vi "HFRR ADV v06.vi"() -> ()   [LabVIEW 2025] (continued)
              n1765 = Fract/Exp String To Number(string=w2180) -> (number=w2183:dbl)  [unwired: 3 in, 1 out]
              n1766 = Add(x=w2183, y=0.0) -> (x+y=w2179:dbl)
            }
            n1767 = for {
              N: w2071 -> [_]
              tunnel: w2078 -> [w2126]
              tunnel: w2077 -> [w2125]
              tunnel: [w2115] -> w2031 mode=indexing
              tunnel: [w2114] -> w2024 mode=indexing
              tunnel: w2068 -> [_]
              tunnel: [w2103] -> w2029 mode=indexing
              tunnel: [w2108] -> w2026 mode=indexing
              tunnel: [w2104] -> w2016 mode=indexing
              tunnel: [w2099] -> w1991 mode=indexing
              tunnel: [w2095] -> w1972 mode=indexing
              tunnel: [w2090] -> w1932 mode=indexing
              (unwired) 1.0 ("x")
              (unwired) TRUE ("line mode (F)")
              n1768 = Read from Text File "Read File"(file (use dialog)=w2126, error in=w2125) -> (text=w2091:string)  [unwired: 2 in, 3 out]
              n1769 = local write "String 12"(w2091) -> ()
              n1770 = String Subset(string=w2091, offset (0)=85, length (rest)=9 ("length (rest)")) -> (substring=w2093:string)
              n1771 = String Subset(string=w2091, offset (0)=35, length (rest)=9 ("length (rest)")) -> (substring=w2116:string)
              n1772 = String Subset(string=w2091, offset (0)=55, length (rest)=9 ("length (rest)")) -> (substring=w2101:string)
              n1773 = String Subset(string=w2091, offset (0)=25, length (rest)=9 ("length (rest)")) -> (substring=w2097:string)
              n1774 = String Subset(string=w2091, offset (0)=45, length (rest)=9 ("length (rest)")) -> (substring=w2106:string)
              n1775 = String Subset(string=w2091, offset (0)=15, length (rest)=9 ("length (rest)")) -> (substring=w2122:string)
              n1776 = String Subset(string=w2091, offset (0)=0, length (rest)=14 ("length (rest)")) -> (substring=w2119:string)
              n1777 = String Subset(string=w2091, offset (0)=65, length (rest)=9 ("length (rest)")) -> (substring=w2109:string)
              n1778 = Fract/Exp String To Number(string=w2093) -> (number=w2090:dbl)  [unwired: 3 in, 1 out]
              n1779 = Fract/Exp String To Number(string=w2116) -> (number=w2114:dbl)  [unwired: 3 in, 1 out]
              n1780 = Fract/Exp String To Number(string=w2101) -> (number=w2099:dbl)  [unwired: 3 in, 1 out]
              n1781 = Fract/Exp String To Number(string=w2097) -> (number=w2095:dbl)  [unwired: 3 in, 1 out]
              n1782 = Fract/Exp String To Number(string=w2106) -> (number=w2104:dbl)  [unwired: 3 in, 1 out]
              n1783 = Fract/Exp String To Number(string=w2122) -> (number=w2103:dbl)  [unwired: 3 in, 1 out]
              n1784 = Fract/Exp String To Number(string=w2119) -> (number=w2115:dbl)  [unwired: 3 in, 1 out]
              n1785 = Fract/Exp String To Number(string=w2109) -> (number=w2112:dbl)  [unwired: 3 in, 1 out]
              n1786 = Add(x=w2112, y=0.0) -> (x+y=w2108:dbl)
            }
            n1787 = Delete From Array(array=w1974, index=0) -> (array with subset deleted=w1947:dbl[])  [unwired: 1 in, 1 out]
            n1788 = Delete From Array(array=w2037, index=0) -> (array with subset deleted=w2010:dbl[])  [unwired: 1 in, 1 out]
            n1789 = Delete From Array(array=w2017, index=0) -> (array with subset deleted=w2005:dbl[])  [unwired: 1 in, 1 out]
            n1790 = Delete From Array(array=w2035, index=0) -> (array with subset deleted=w2036:dbl[])  [unwired: 1 in, 1 out]
            n1791 = call-poly <vilib>:"Mean.vi"("X"=w1947) -> ("mean"=→"КОФ2 4":dbl)  [unwired: 1 out]
            n1792 = call-poly <vilib>:"Mean.vi"("X"=w2010) -> ("mean"=→"КОФ3":dbl)  [unwired: 1 out]
            n1793 = call-poly <vilib>:"Mean.vi"("X"=w2005) -> ("mean"=→"CP3":dbl)  [unwired: 1 out]
            n1794 = Delete From Array(array=w1999, index=0) -> (array with subset deleted=w1926:dbl[])  [unwired: 1 in, 1 out]
            n1795 = Delete From Array(array=w1938, index=0) -> (array with subset deleted=w1925:dbl[])  [unwired: 1 in, 1 out]
            n1796 = Delete From Array(array=w1978, index=0) -> (array with subset deleted=w1949:dbl[])  [unwired: 1 in, 1 out]
            n1797 = Delete From Array(array=w2056, index=0) -> (array with subset deleted=w2011:dbl[])  [unwired: 1 in, 1 out]
            n1798 = Delete From Array(array=w2022, index=0) -> (array with subset deleted=w2007:dbl[])  [unwired: 1 in, 1 out]
            "array w/ subset deleted" <- w2007
            n1799 = Delete From Array(array=w2053, index=0) -> (array with subset deleted=w2054:dbl[])  [unwired: 1 in, 1 out]
            n1800 = call-poly <vilib>:"Mean.vi"("X"=w1949) -> ("mean"=→"КОФ2 2":dbl)  [unwired: 1 out]
            n1801 = call-poly <vilib>:"Mean.vi"("X"=w2011) -> ("mean"=→"КОФ1":dbl)  [unwired: 1 out]
            n1802 = Bundle "Bundle"(w1926, w1925) -> (w1931:cluster{dbl[], dbl[]})  [unwired: 1 in]
            n1803 = Bundle "Bundle"(w1926, w2054) -> (w1918:cluster{dbl[], dbl[]})  [unwired: 1 in]
            n1804 = Delete From Array(array=w1933, index=0) -> (array with subset deleted=w1921:dbl[])  [unwired: 1 in, 1 out]
            n1805 = Delete From Array(array=w1934, index=0) -> (array with subset deleted=w1923:dbl[])  [unwired: 1 in, 1 out]
            n1806 = Delete From Array(array=w2044, index=0) -> (array with subset deleted=w2045:dbl[])  [unwired: 1 in, 1 out]
            n1807 = Delete From Array(array=w1932, index=0) -> (array with subset deleted=w1919:dbl[])  [unwired: 1 in, 1 out]
            n1808 = Delete From Array(array=w2026, index=0) -> (array with subset deleted=w2027:dbl[])  [unwired: 1 in, 1 out]
            n1809 = Delete From Array(array=w2051, index=0) -> (array with subset deleted=w1957:dbl[])  [unwired: 1 in, 1 out]
            n1810 = Delete From Array(array=w1997, index=0) -> (array with subset deleted=w1953:dbl[])  [unwired: 1 in, 1 out]
            n1811 = Delete From Array(array=w2033, index=0) -> (array with subset deleted=w1955:dbl[])  [unwired: 1 in, 1 out]
            n1812 = Delete From Array(array=w1993, index=0) -> (array with subset deleted=w1951:dbl[])  [unwired: 1 in, 1 out]
            n1813 = Delete From Array(array=w2042, index=0) -> (array with subset deleted=w1956:dbl[])  [unwired: 1 in, 1 out]
            n1814 = Delete From Array(array=w1995, index=0) -> (array with subset deleted=w1952:dbl[])  [unwired: 1 in, 1 out]
            n1815 = Delete From Array(array=w1976, index=0) -> (array with subset deleted=w1948:dbl[])  [unwired: 1 in, 1 out]
            n1816 = Delete From Array(array=w2020, index=0) -> (array with subset deleted=w2006:dbl[])  [unwired: 1 in, 1 out]
            n1817 = Delete From Array(array=w2047, index=0) -> (array with subset deleted=w2008:dbl[])  [unwired: 1 in, 1 out]
            n1818 = Delete From Array(array=w2024, index=0) -> (array with subset deleted=w1954:dbl[])  [unwired: 1 in, 1 out]
            n1819 = Delete From Array(array=w1991, index=0) -> (array with subset deleted=w1950:dbl[])  [unwired: 1 in, 1 out]
            n1820 = Delete From Array(array=w1972, index=0) -> (array with subset deleted=w1946:dbl[])  [unwired: 1 in, 1 out]
            n1821 = Delete From Array(array=w2016, index=0) -> (array with subset deleted=w2004:dbl[])  [unwired: 1 in, 1 out]
            n1822 = Delete From Array(array=w2029, index=0) -> (array with subset deleted=w2009:dbl[])  [unwired: 1 in, 1 out]
            n1823 = Delete From Array(array=w2039, index=0) -> (array with subset deleted=w1922:dbl[])  [unwired: 1 in, 1 out]
            n1824 = Delete From Array(array=w2049, index=0) -> (array with subset deleted=w1924:dbl[])  [unwired: 1 in, 1 out]
            n1825 = Delete From Array(array=w2031, index=0) -> (array with subset deleted=w1920:dbl[])  [unwired: 1 in, 1 out]
            n1826 = Bundle "Bundle"(w1926, w1957) -> (w1944:cluster{dbl[], dbl[]})  [unwired: 1 in]
            n1827 = Bundle "Bundle"(w1926, w2011) -> (w1945:cluster{dbl[], dbl[]})  [unwired: 1 in]
            n1828 = Bundle "Bundle"(w1957, w1953) -> (w1959:cluster{dbl[], dbl[]})  [unwired: 1 in]
            n1829 = Bundle "Bundle"(w1922, w1921) -> (w1929:cluster{dbl[], dbl[]})  [unwired: 1 in]
            n1830 = Bundle "Bundle"(w1955, w1951) -> (w1961:cluster{dbl[], dbl[]})  [unwired: 1 in]
            n1831 = Bundle "Bundle"(w1922, w1955) -> (w2065:cluster{dbl[], dbl[]})  [unwired: 1 in]
            n1832 = Bundle "Bundle"(w1922, w1951) -> (w1989:cluster{dbl[], dbl[]})  [unwired: 1 in]
            n1833 = Bundle "Bundle"(w1922, w2010) -> (w2075:cluster{dbl[], dbl[]})  [unwired: 1 in]
            n1834 = Bundle "Bundle"(w1922, w2005) -> (w2013:cluster{dbl[], dbl[]})  [unwired: 1 in]
            n1835 = Bundle "Bundle"(w1922, w2036) -> (w2060:cluster{dbl[], dbl[]})  [unwired: 1 in]
            n1836 = Bundle "Bundle"(w1956, w1952) -> (w1960:cluster{dbl[], dbl[]})  [unwired: 1 in]
            n1837 = Bundle "Bundle"(w1924, w1923) -> (w1930:cluster{dbl[], dbl[]})  [unwired: 1 in]
            n1838 = Bundle "Bundle"(w1924, w1956) -> (w2067:cluster{dbl[], dbl[]})  [unwired: 1 in]
            n1839 = Bundle "Bundle"(w1924, w1952) -> (w1990:cluster{dbl[], dbl[]})  [unwired: 1 in]
            n1840 = Bundle "Bundle"(w1924, w2006) -> (w2014:cluster{dbl[], dbl[]})  [unwired: 1 in]
            n1841 = Bundle "Bundle"(w1924, w2008) -> (w2076:cluster{dbl[], dbl[]})  [unwired: 1 in]
            n1842 = Bundle "Bundle"(w1924, w2045) -> (w2058:cluster{dbl[], dbl[]})  [unwired: 1 in]
            n1843 = Bundle "Bundle"(w1954, w1950) -> (w1962:cluster{dbl[], dbl[]})  [unwired: 1 in]
            n1844 = Bundle "Bundle"(w1920, w1919) -> (w1928:cluster{dbl[], dbl[]})  [unwired: 1 in]
            n1845 = Bundle "Bundle"(w1920, w1954) -> (w2066:cluster{dbl[], dbl[]})  [unwired: 1 in]
            n1846 = Bundle "Bundle"(w1920, w1950) -> (w1988:cluster{dbl[], dbl[]})  [unwired: 1 in]
            n1847 = Bundle "Bundle"(w1920, w2004) -> (w2012:cluster{dbl[], dbl[]})  [unwired: 1 in]
            n1848 = Bundle "Bundle"(w1920, w2009) -> (w2074:cluster{dbl[], dbl[]})  [unwired: 1 in]
            n1849 = Bundle "Bundle"(w1920, w2027) -> (w2059:cluster{dbl[], dbl[]})  [unwired: 1 in]
            n1850 = call-poly <vilib>:"Mean.vi"("X"=w2007) -> ("mean"=→"CP1":dbl)  [unwired: 1 out]
            n1851 = call-poly <vilib>:"Mean.vi"("X"=w1948) -> ("mean"=→"КОФ2 3":dbl)  [unwired: 1 out]
            n1852 = call-poly <vilib>:"Mean.vi"("X"=w2006) -> ("mean"=→"CP2":dbl)  [unwired: 1 out]
            n1853 = call-poly <vilib>:"Mean.vi"("X"=w2008) -> ("mean"=→"КОФ2":dbl)  [unwired: 1 out]
            n1854 = call-poly <vilib>:"Mean.vi"("X"=w1946) -> ("mean"=→"КОФ2 5":dbl)  [unwired: 1 out]
            n1855 = call-poly <vilib>:"Mean.vi"("X"=w2004) -> ("mean"=→"CP4":dbl)  [unwired: 1 out]
            n1856 = call-poly <vilib>:"Mean.vi"("X"=w2009) -> ("mean"=→"КОФ4":dbl)  [unwired: 1 out]
            n1857 = Bundle "Bundle"(w1926, w1953) -> (w1917:cluster{dbl[], dbl[]})  [unwired: 1 in]
            n1858 = Bundle "Bundle"(w1926, w2007) -> (w1940:cluster{dbl[], dbl[]})  [unwired: 1 in]
            n1859 = Build Array "Build Array"(w1917, w1940) -> (w1943:cluster{dbl[], dbl[]}[])
            "XY Graph 17" <- w1943
            n1860 = Build Array "Build Array"(w1931, w1930, w1929, w1928) -> (→"Frequency ( Hz )":cluster{dbl[], dbl[]}[])
            n1861 = Build Array "Build Array"(w1959, w1960, w1961, w1962) -> (→"Air Temp ( °C ) vs Humidity ( % Rh )":cluster{dbl[], dbl[]}[])
            n1862 = Build Array "Build Array"(w1944, w2067, w2065, w2066) -> (→"Air Temperature  ( °C )":cluster{dbl[], dbl[]}[])
            n1863 = Build Array "Build Array"(w1917, w1990, w1989, w1988) -> (→"Humidity ( %Rh )":cluster{dbl[], dbl[]}[])
            n1864 = Build Array "Build Array"(w1945, w2076, w2075, w2074) -> (→"Coefficient Of Friction":cluster{dbl[], dbl[]}[])
            n1865 = Build Array "Build Array"(w1940, w2014, w2013, w2012) -> (→"Sample Temperature ( °C )":cluster{dbl[], dbl[]}[])
            n1866 = Build Array "Build Array"(w1918, w2058, w2060, w2059) -> (→"XY Graph 13":cluster{dbl[], dbl[]}[])
            n1867 = Bundle "Bundle"(w1926, w1949) -> (w1971:cluster{dbl[], dbl[]})  [unwired: 1 in]
            n1868 = Bundle "Bundle"(w1922, w1947) -> (w1969:cluster{dbl[], dbl[]})  [unwired: 1 in]
            n1869 = Bundle "Bundle"(w1924, w1948) -> (w1970:cluster{dbl[], dbl[]})  [unwired: 1 in]
            n1870 = Bundle "Bundle"(w1920, w1946) -> (w1968:cluster{dbl[], dbl[]})  [unwired: 1 in]
            n1871 = Build Array "Build Array"(w1971, w1970, w1969, w1968) -> (→"Stroke ( mm )":cluster{dbl[], dbl[]}[])
            n1872 = local write "XY Graph 16"(w1943) -> ()
          }
          frame #2 {
          }
          frame #3 {
            n1873 = local write "Numeric 8"(0 ("Numeric 8")) -> ()
            n1874 = local write "Numeric 11"(0 ("Numeric 11")) -> ()
            n1875 = local write "Numeric 12"(0 ("Numeric 12")) -> ()
            n1876 = local write "Numeric 13"(0 ("Numeric 13")) -> ()
            n1877 = property on="OPEN" class="Bool (strict)"("Visible"=TRUE) -> ()  [unwired: 2 in, 2 out]
            n1878 = local read "String Control 2"() -> (w2243:string)
            n1879 = local read "String Control 4"() -> (w2242:string)
            n1880 = local read "String Control 6"() -> (w2241:string)
            n1881 = local read "String Control 8"() -> (w2240:string)
            n1882 = Match Pattern(string=w2243, regular expression="Samples / cycle :- ") -> (after substring=w2257:string)  [unwired: 1 in, 3 out]
            n1883 = Match Pattern(string=w2243, regular expression="Frequency :- ") -> (after substring=w2276:string)  [unwired: 1 in, 3 out]
            n1884 = Match Pattern(string=w2242, regular expression="Samples / cycle :- ") -> (after substring=w2253:string)  [unwired: 1 in, 3 out]
            n1885 = Match Pattern(string=w2242, regular expression="Frequency :- ") -> (after substring=w2271:string)  [unwired: 1 in, 3 out]
            n1886 = Match Pattern(string=w2241, regular expression="Samples / cycle :- ") -> (after substring=w2249:string)  [unwired: 1 in, 3 out]
            n1887 = Match Pattern(string=w2241, regular expression="Frequency :- ") -> (after substring=w2266:string)  [unwired: 1 in, 3 out]
            n1888 = Match Pattern(string=w2240, regular expression="Samples / cycle :- ") -> (after substring=w2245:string)  [unwired: 1 in, 3 out]
            n1889 = Match Pattern(string=w2240, regular expression="Frequency :- ") -> (after substring=w2261:string)  [unwired: 1 in, 3 out]
            n1890 = String Subset(string=w2257, length (rest)=6 ("length (rest)")) -> (substring=w2259:string)  [unwired: 1 in]
            n1891 = String Subset(string=w2276, length (rest)=9 ("length (rest)")) -> (substring=w2278:string)  [unwired: 1 in]
            n1892 = String Subset(string=w2253, length (rest)=6 ("length (rest)")) -> (substring=w2255:string)  [unwired: 1 in]
            n1893 = String Subset(string=w2271, length (rest)=9 ("length (rest)")) -> (substring=w2273:string)  [unwired: 1 in]
            n1894 = String Subset(string=w2249, length (rest)=6 ("length (rest)")) -> (substring=w2251:string)  [unwired: 1 in]
            n1895 = String Subset(string=w2266, length (rest)=9 ("length (rest)")) -> (substring=w2268:string)  [unwired: 1 in]
            n1896 = String Subset(string=w2245, length (rest)=6 ("length (rest)")) -> (substring=w2247:string)  [unwired: 1 in]
            n1897 = String Subset(string=w2261, length (rest)=9 ("length (rest)")) -> (substring=w2263:string)  [unwired: 1 in]
            n1898 = Fract/Exp String To Number(string=w2259) -> (number=w2239:dbl)  [unwired: 3 in, 1 out]
            n1899 = Fract/Exp String To Number(string=w2278) -> (number=w2279:dbl)  [unwired: 3 in, 1 out]
            n1900 = Fract/Exp String To Number(string=w2255) -> (number=w2238:dbl)  [unwired: 3 in, 1 out]
            n1901 = Fract/Exp String To Number(string=w2273) -> (number=w2274:dbl)  [unwired: 3 in, 1 out]
            n1902 = Fract/Exp String To Number(string=w2251) -> (number=w2237:dbl)  [unwired: 3 in, 1 out]
            n1903 = Fract/Exp String To Number(string=w2268) -> (number=w2269:dbl)  [unwired: 3 in, 1 out]
            n1904 = Fract/Exp String To Number(string=w2247) -> (number=w2236:dbl)  [unwired: 3 in, 1 out]
            n1905 = Fract/Exp String To Number(string=w2263) -> (number=w2264:dbl)  [unwired: 3 in, 1 out]
            n1906 = local write "sample1"(w2239) -> ()
            n1907 = local write "freq1"(w2279) -> ()
            n1908 = local write "sample2"(w2238) -> ()
            n1909 = local write "freq2"(w2274) -> ()
            n1910 = local write "sample3"(w2237) -> ()
            n1911 = local write "freq3"(w2269) -> ()
            n1912 = local write "sample4"(w2236) -> ()
            n1913 = local write "freq 4"(w2264) -> ()
          }
        }
      }
    }
    n1914 = case shown="True" w1727 {
      selector: w1727 -> [_ w1856]
      frame False {
      }
      frame True {
        n1915 = Not(x=w1856) -> (.not. x?=w1852:bool)
        n1916 = local write "service 3"(w1852) -> ()
        n1917 = local write "OPEN 6"(w1852) -> ()
        n1918 = call <vilib>:"System Exec.vi"("wait until completion? (T)"=TRUE, "command line"="C:\\LAB-IQ\\Scar View.exe") -> ("error out"=→"error out 5":errorcluster)  [unwired: 6 in, 3 out]
      }
    }
    n1919 = case shown="\"About\"" w1739 {
      frame "Acquire", Default {
        w2760 = 0.2 ("y")
        w2765 = 1.0 ("y")
        w2766 = 0.8 ("y")
        # "Elapsed time\ncof\nstroke\nAir temp\nTemp\nHumidity"
        n1920 = disable-structure shown="Disabled" {
          frame Disabled {
            n1921 = local read "Flag"() -> (w2783:dbl)
            n1922 = local read "RUN"() -> (w2780:bool)
            n1923 = Not(x=w2780) -> (.not. x?=w2779:bool)
            n1924 = Equal?(x=w2783, y=10.0) -> (x = y?=w2781:bool)
            n1925 = And(x=w2781, y=w2779) -> (x .and. y?=w2778:bool)
            n1926 = case shown="True" w2778 {
              frame False {
              }
              frame True {
                w2784 = FALSE ("Heater Button")
                n1927 = local write "Humidity"(w2784) -> ()
                n1928 = local write "Heater Button"(w2784) -> ()
              }
            }
          }
          frame Enabled {
          }
        }
        n1929 = disable-structure shown="Disabled" {
          frame Disabled {
            n1930 = case shown="True" {
              selector: _ -> [_ _]
              frame False {
              }
              frame True {
                w2875 = TRUE ("Heater")
                n1931 = local write "Humidity"(w2875) -> ()
                n1932 = local write "Heater Button"(w2875) -> ()
                n1933 = local read "TEST STANDARD"() -> (w2878:T3)
                n1934 = local read "TEST STANDARD"() -> (w2873:T3)
                n1935 = Equal?(x=w2878, y=enum16{"ASTM D6079", "ISO 12156", "Custom"}."ISO 12156" ("Test Standard")) -> (x = y?=w2876:bool)
                n1936 = Equal?(x=w2873, y=enum16{"ASTM D6079", "ISO 12156", "Custom"}."ASTM D6079" ("Test Standard")) -> (x = y?=w2872:bool)
                n1937 = case shown="True" w2876 {
                  frame False {
                  }
                  frame True {
                    n1938 = local write "Heater"(TRUE ("Heater")) -> ()
                    n1939 = local write "airtempflg"(FALSE ("airtempflg")) -> ()
                  }
                }
                n1940 = case shown="True" w2872 {
                  frame False {
                  }
                  frame True {
                    n1941 = local write "Heater"(FALSE ("Heater")) -> ()
                    n1942 = local write "airtempflg"(TRUE ("airtempflg")) -> ()
                  }
                }
              }
            }
          }
          frame Enabled {
          }
        }
        n1943 = stacked-sequence {
          frame #0 {
            n1944 = case shown="True" "RST FF" {
              frame False {
              }
              frame True {
                w2941 = 0.0 ("X Scale.Range:Maximum")
                n1945 = property on="Frictional Force ( N )" class="WFChart (strict)"("XScale.Maximum"=600.0 ("X Scale.Range:Maximum"), "XScale.Minimum"=w2941, "YScale.Maximum"=10.0 ("Y Scale.Range:Maximum"), "YScale.Minimum"=w2941) -> ()  [unwired: 2 in, 2 out]
              }
            }
          }
          frame #1 {
            n1946 = case shown="True" "RST TEMP" {
              frame False {
              }
              frame True {
                n1947 = property on="Temperature ( Deg C )" class="WFChart (strict)"("XScale.Minimum"=0.0 ("X Scale.Range:Minimum"), "XScale.Maximum"=600.0 ("X Scale.Range:Maximum"), "YScale.Minimum"=0.0 ("Y Scale.Range:Minimum"), "YScale.Maximum"=100.0 ("Y Scale.Range:Maximum")) -> ()  [unwired: 2 in, 2 out]
              }
            }
          }
          frame #2 {
            n1948 = case shown="True" "RSTCOF" {
              frame False {
              }
              frame True {
                n1949 = property on="Coefficient of Friction" class="WFChart (strict)"("XScale.Minimum"=0.0 ("X Scale.Range:Minimum"), "XScale.Maximum"=600.0 ("X Scale.Range:Maximum"), "YScale.Maximum"=1.0 ("X Scale.Range:Minimum"), "YScale.Minimum"=0.0 ("X Scale.Range:Minimum")) -> ()  [unwired: 2 in, 2 out]
              }
            }
          }
          frame #3 {
            n1950 = case shown="True" "RSTCOF 2" {
              frame False {
              }
              frame True {
                (unwired) 100.0 ("Y Scale.Range:Maximum")
                (unwired) 0.0 ("Y Scale.Range:Minimum")
                (unwired) 600.0 ("X Scale.Range:Maximum")
                (unwired) 0.0 ("X Scale.Range:Minimum")
              }
            }
          }
          frame #4 {
            n1951 = case shown="True" "RSTCOF 3" {
              frame False {
              }
              frame True {
                n1952 = property on="Electrical Contact Resistance ( % )" class="WFChart (strict)"("XScale.Minimum"=0.0 ("X Scale.Range:Minimum"), "XScale.Maximum"=600.0 ("X Scale.Range:Maximum"), "YScale.Minimum"=0.0 ("Y Scale.Range:Minimum"), "YScale.Maximum"=100.0 ("Y Scale.Range:Maximum")) -> ()  [unwired: 2 in, 2 out]
              }
            }
          }
        }
        n1953 = disable-structure shown="Disabled" {
          frame Disabled {
            n1954 = case shown="True" {
              selector: _ -> [_ _]
              frame False {
              }
              frame True {
                n1955 = local read "zflag 2"() -> (w2842:dbl)
                n1956 = local read "yflag"() -> (w2844:dbl)
                n1957 = Equal?(x=w2844, y=2.0 ("tflag")) -> (x = y?=w2846:bool)
                n1958 = Equal?(x=w2842, y=3.0 ("tflag")) -> (x = y?=w2845:bool)
                n1959 = And(x=w2846, y=w2845) -> (x .and. y?=w2840:bool)
                n1960 = case shown="True" w2840 {
                  frame False {
                  }
                  frame True {
                    w2871 = 0.0 ("zflag")
                    n1961 = local write "zflag"(w2871) -> ()
                    n1962 = local write "zflag 2"(w2871) -> ()
                    n1963 = Delete(path (use dialog)=path "C:/LAB-IQ-NXT/WO 2449 TT.sig" ("file path (dialog if empty)")) -> (deleted path=w2870:path)  [unwired: 4 in, 2 out]
                    n1964 = Delete(path (use dialog)=path "C:/LAB-IQ-NXT/WO 2449 TRH.sig" ("file path (dialog if empty)")) -> (deleted path=w2865:path)  [unwired: 4 in, 2 out]
                    n1965 = local read "SEN.RUN HRS"() -> (w2857:dbl)
                    n1966 = local read "SENSOR TIME"() -> (w2855:dbl)
                    n1967 = call <vilib>:"compatOverwrite.vi"("overwrite (F)"=TRUE) -> ("overwrite?"=w2847:T21)
                    n1968 = call <vilib>:"compatOverwrite.vi"("overwrite (F)"=TRUE) -> ("overwrite?"=w2851:T21)
                    n1969 = local read "Total No. of Tests"() -> (w2858:dbl)
                    n1970 = Add(x=w2855, y=w2857) -> (x+y=w2856:dbl)
                    "SEN.RUN HRS" <- w2856
                    n1971 = Open/Create/Replace File(file path (use dialog)=w2870, operation (0:open)=w2847) -> (refnum out=w2848:refnum<file>, error out=w2849:errorcluster)  [unwired: 4 in, 1 out]
                    n1972 = Open/Create/Replace File(file path (use dialog)=w2865, operation (0:open)=w2851) -> (refnum out=w2852:refnum<file>, error out=w2853:errorcluster)  [unwired: 4 in, 1 out]
                    n1973 = Deny Access(4:w2849, 6:T19."deny none" ("deny mode (2)"), 7:w2848) -> (3:w2869:refnum<file>)  [unwired: 1 out]
                    n1974 = Deny Access(4:w2853, 6:T19."deny none" ("deny mode (2)"), 7:w2852) -> (3:w2861:refnum<file>)  [unwired: 1 out]
                    n1975 = Number To Decimal String(number=w2858) -> (decimal integer string=w2866:string)  [unwired: 1 in]
                    n1976 = Number To Decimal String(number=w2856) -> (decimal integer string=w2862:string)  [unwired: 1 in]
                    n1977 = Write to Binary File(file (use dialog)=w2869, data=w2866, 5:FALSE ("prepend array or string size? (T)")) -> ()  [unwired: 3 in, 3 out]
                    n1978 = Write to Binary File(file (use dialog)=w2861, data=w2862, 5:FALSE ("prepend array or string size? (T)")) -> ()  [unwired: 3 in, 3 out]
                  }
                }
              }
            }
          }
          frame Enabled {
          }
        }
        n1979 = local read "RUN"() -> (w2769:bool)
        n1980 = local read "run replace"() -> (w2773:bool)
        n1981 = local read "run replace"() -> (w2772:bool)
        n1982 = case shown="True" w2769 {
          frame False {
            n1983 = local write "run replace"(FALSE ("run replace")) -> ()
          }
          frame True {
            "run replace" <- TRUE ("run replace")
          }
        }
        n1984 = local read "RUN"() -> (w2777:bool)
        n1985 = local read "Set Temp"() -> (w2739:dbl)
        n1986 = local read "SetTemp"() -> (w2741:dbl)
        n1987 = case shown="False" w2777 {
          tunnel: [FALSE ("TEST RUNNING") TRUE ("TEST RUNNING")] -> w2776
          frame False {
            w2960 = 0.0 ("Flag")
            n1988 = local write "Elapsed time"(0.0 ("elapsedtime")) -> ()
            n1989 = local write "Time Remaining"(w2960) -> ()
            n1990 = local write "Flag"(w2960) -> ()
          }
          frame True {
            n1991 = local write "Flag"(10.0 ("Flag")) -> ()
          }
        }
        n1992 = case shown="False" w2773 {
          frame False {
            n1993 = local read "zflag"() -> (→"zflag 2":dbl)
            n1994 = local write "yflag"(2.0 ("tflag")) -> ()
            n1995 = local write "FLAG 4"(0.0 ("FLAG")) -> ()
          }
          frame True {
            n1996 = local write "yflag"(1.0 ("tflag")) -> ()
            n1997 = local write "zflag"(3.0 ("zflag")) -> ()
          }
        }
        n1998 = local read "acq 2"() -> (w2771:bool)
        n1999 = local read "AIR TEMP"() -> (w2734:dbl)
        n2000 = local read "Amb temp"() -> (w2738:dbl)
        n2001 = case shown="True" "Save & Continue" {
          frame False {
          }
          frame True {
            "acq 2" <- TRUE ("acq 2")
          }
        }
        n2002 = case shown="True" "Save & Continue" {
          frame False {
          }
          frame True {
            n2003 = while {
              tunnel: "0123456789abcdefghijklmnopqrstuvwxyzABCDEFGHIJKLMNOPQRSTUVWXYZ" ("string 2") -> [w2931]
              shift-right: [w2929] -> w2924
              shift-left: "" -> [w2928]
              i -> [w2938]
              stop <- w2937 stop-if-true
              n2004 = Random Number (0-1)() -> (number: 0 to 1=w2932:dbl)
              n2005 = Multiply(x=w2932, y=62.0) -> (x*y=w2934:dbl)
              n2006 = Decrement(x="Length") -> (x-1=w2927:i16)
              n2007 = To Word Integer(number=w2934) -> (16bit integer=w2935:i16)
              n2008 = String Subset(string=w2931, offset (0)=w2935, length (rest)=1 ("length (rest)")) -> (substring=w2930:string)
              n2009 = Greater Or Equal?(x=w2938, y=w2927) -> (x >= y?=w2937:bool)
              n2010 = Concatenate Strings(w2930, w2928) -> (w2929:string)
            }
            n2011 = local write "UUID"(w2924) -> ()
          }
        }
        n2012 = case shown="True" "Save & Continue" {
          frame False {
          }
          frame True {
            n2013 = local read "Operator ID"() -> (w3220:string)
            n2014 = local read "FILE"() -> (w3226:string)
            n2015 = String Length(string=w3226) -> (length=w3224:i32)
            n2016 = String Length(string=w3220) -> (length=w3221:i32)
            n2017 = Greater?(x=w3224, y=0) -> (0:w3223:bool)
            n2018 = Greater?(x=w3221, y=0) -> (0:w3219:bool)
            n2019 = And(x=w3223, y=w3219) -> (x .and. y?=w3218:bool)
            n2020 = case shown="True" w3218 {
              frame False {
                n2021 = stacked-sequence {
                  frame #0 {
                    n2022 = One Button Dialog(message="Please Enter a File Name and Operator ID to save data !", button name ("OK")="Ok") -> ()  [unwired: 1 out]
                  }
                  frame #1 {
                    n2023 = local write "Save & Continue"(FALSE ("OK Button")) -> ()
                  }
                }
                n2024 = local write "Save & Continue"(FALSE ("OK Button")) -> ()
              }
              frame True {
                n2025 = stacked-sequence {
                  frame #0 {
                    n2026 = call <vilib>:"Application Directory.vi"() -> ("Application Directory"=w3234:path)
                    n2027 = Build Path(base path=w3234, name or relative path="data") -> (appended path=w3233:path)
                    n2028 = local read "FILE"() -> (w3236:string)
                    n2029 = List Folder(path=w3233) -> (folder names=w3232:string[])  [unwired: 3 in, 3 out]
                    n2030 = Equal?(x=w3232, y=w3236) -> (x = y?=w3238:bool[])
                    n2031 = call <vilib>:"Trim Whitespace.vi"("string"=w3236) -> ("trimmed string"=w3231:string)  [unwired: 1 in]
                    n2032 = Or Array Elements(Boolean array=w3238) -> (logical OR=w3237:bool)
                    n2033 = case shown="True" w3237 {
                      tunnel: w3231 -> [_ w3240]
                      frame False {
                      }
                      frame True {
                        w3243 = "_(" ("regular expression")
                        n2034 = Match Pattern(string=w3240, regular expression=w3243) -> (match substring=w3242:string, after substring=w3239:string)  [unwired: 1 in, 2 out]
                        n2035 = Equal?(x=w3242, y=w3243) -> (x = y?=w3241:bool)
                        n2036 = case shown="False" w3241 {
                          tunnel: w3240 -> [w3246 w3256]
                          tunnel: w3239 -> [_ w3258]
                          frame False {
                            n2037 = Concatenate Strings(w3246, "_(" ("regular expression"), "1" ("string"), ")" ("regular expression")) -> (w3244:string)
                            n2038 = local write "FILE"(w3244) -> ()
                          }
                          frame True {
                            n2039 = Decimal String To Number(string=w3258) -> (number=w3257:i32)  [unwired: 2 in, 1 out]
                            n2040 = Search/Split String(string=w3256, search string/char (-)="_(" ("regular expression")) -> (substring before match=w3254:string)  [unwired: 1 in, 2 out]
                            n2041 = Increment(x=w3257) -> (x+1=w3252:i32)
                            n2042 = Number To Decimal String(number=w3252) -> (decimal integer string=w3251:string)  [unwired: 1 in]
                            n2043 = Concatenate Strings(w3254, "_(" ("regular expression"), w3251, ")" ("regular expression")) -> (w3249:string)
                            n2044 = local write "FILE"(w3249) -> ()
                          }
                        }
                      }
                    }
                  }
                  frame #1 {
                    w3269 = 0.0
                    w3271 = cluster{"y":dbl, dbl, "y":dbl}[] [] ("History Data")
                    w3272 = FALSE ("Heater Button")
                    (unwired) ")!" ("string")
                    (unwired) ")" ("string")
                    w3270 = dbl[] [] ("History Data")
                    w3276 = "\r"
                    # "C:\\WinDucom\\Data\\"
                    # "C:\\LAB-IQ-NXT\\data"
                    n2045 = local write "Humidity ( %RH )"(w3269) -> ()
                    n2046 = local write "Frequency ( Hz )"(w3269) -> ()
                    n2047 = local write "speedop"(0.0 ("PIDclk 2")) -> ()
                    n2048 = local write "Set Temp 2"(w3269) -> ()
                    n2049 = local write "AIR TEMP"(w3269) -> ()
                    n2050 = local write "clk"(0.0 ("clk")) -> ()
                    n2051 = local write "Stroke 4"(w3269) -> ()
                    n2052 = local write "Stroke"(w3269) -> ()
                    n2053 = local write "COF 3"(w3269) -> ()
                    n2054 = local write "COF 2"(w3269) -> ()
                    n2055 = local write "TEMP"(w3269) -> ()
                    n2056 = local write "ecr 3"(w3269) -> ()
                    n2057 = local write "FF 3"(w3269) -> ()
                    n2058 = local write "FF 2"(w3269) -> ()
                    n2059 = property on="Humidity ( %RH )" class="WFChart (strict)"("History Data"=w3270) -> ()  [unwired: 2 in, 2 out]
                    n2060 = property on="Coefficient of Friction" class="WFChart (strict)"("History Data"=w3270) -> ()  [unwired: 2 in, 2 out]
                    n2061 = property on="Coefficient of Friction" class="WFChart (strict)"("History Data"=w3270) -> ()  [unwired: 2 in, 2 out]
                    n2062 = property on="Frictional Force ( N )" class="WFChart (strict)"("History Data"=w3270) -> ()  [unwired: 2 in, 2 out]
                    n2063 = property on="Electrical Contact Resistance ( % )" class="WFChart (strict)"("History Data"=w3270) -> ()  [unwired: 2 in, 2 out]
                    n2064 = property on="Electrical Contact Resistance ( % )" class="WFChart (strict)"("History Data"=w3270) -> ()  [unwired: 2 in, 2 out]
                    n2065 = property on="Temperature ( Deg C )" class="WFChart (strict)"("History Data"=w3270) -> ()  [unwired: 2 in, 2 out]
                    n2066 = property on="Frictional Force ( N )" class="WFChart (strict)"("History Data"=w3270) -> ()  [unwired: 2 in, 2 out]
                    n2067 = property on="Coefficient of Friction" class="WFChart (strict)"("History Data"=w3270) -> ()  [unwired: 2 in, 2 out]
                    n2068 = property on="Frictional Force ( N )" class="WFChart (strict)"("History Data"=w3270) -> ()  [unwired: 2 in, 2 out]
                    n2069 = property on="Electrical Contact Resistance ( % )" class="WFChart (strict)"("History Data"=w3270) -> ()  [unwired: 2 in, 2 out]
                    n2070 = property on="Temperature ( Deg C )" class="WFChart (strict)"("History Data"=w3270) -> ()  [unwired: 2 in, 2 out]
                    n2071 = property on="Humidity ( %RH )" class="WFChart (strict)"("History Data"=w3270) -> ()  [unwired: 2 in, 2 out]
                    n2072 = property on="Stroke ( mm )" class="WFChart (strict)"("History Data"=w3271) -> ()  [unwired: 2 in, 2 out]
                    n2073 = property on="Stroke ( mm )" class="WFChart (strict)"("History Data"=w3271) -> ()  [unwired: 2 in, 2 out]
                    n2074 = local write "Humidity"(w3272) -> ()
                    n2075 = local write "Heater Button"(w3272) -> ()
                    n2076 = local read "FILE"() -> (w3265:string)
                    n2077 = local read "NORMAL LOAD"() -> (w3291:dbl)
                    n2078 = call "file check.vi"("file name in"=w3265) -> ("error out"=w3268:errorcluster, "file name out"=w3262:string)  [unwired: 9 in]
                    n2079 = call "FILE PATH CREATION.vi"("error in"=w3268, "FILE NAME :"=w3262) -> ("FILE OUT"=w3261:path)  [unwired: 8 in, 1 out]
                    n2080 = Concatenate Strings(w3262, ".dgf" ("Substring")) -> (w3267:string)
                    n2081 = Concatenate Strings(w3262, ".duf" ("Substring")) -> (w3263:string)
                    n2082 = Multiply(x=w3291, y=1.0) -> (x*y=w3290:dbl)
                    n2083 = Build Path(base path=w3261, name or relative path=w3267) -> (appended path=w3260:path)
                    n2084 = Build Path(base path=w3261, name or relative path=w3263) -> (appended path=w3259:path)
                    n2085 = Number To Fractional String(number=w3290, width (-)=i16 5, precision (6)=i16 2) -> (F-format string=w3299:string)  [unwired: 1 in]
                    n2086 = local read "Fuel Discription :"() -> (w3286:string)
                    n2087 = local read "Batch Ref Num :"() -> (w3274:string)
                    n2088 = Get Date/Time String(date format (0)=enum16{"short", "long", "abbreviated"}."short") -> (date string=w3310:string, time string=w3307:string)  [unwired: 2 in]
                    n2089 = local read "Remarks :"() -> (w3285:string)
                    n2090 = Concatenate Strings("Load :- " ("Substring"), w3299, " N ," ("Substring")) -> (w3298:string)
                    n2091 = local read "String 41"() -> (w3277:string)
                    n2092 = Concatenate Strings(w3286) -> (w3287:string)
                    n2093 = Concatenate Strings(w3274) -> (w3273:string)
                    n2094 = Concatenate Strings("tested by") -> (w3281:string)
                    n2095 = Concatenate Strings("(" ("Substring"), w3310, ")" ("Substring"), w3307) -> (w3279:string)
                    "concatenated string" <- w3279
                    n2096 = Concatenate Strings(w3285, "," ("string")) -> (w3284:string)
                    n2097 = Concatenate Strings("  TIME;      COF;       STROKE;     AIR TEMP;  TEMP;  HUMIDITY;  ECR; PID-OUT; FREQUENCY" ("Substring"), "\r") -> (w3294:string)
                    n2098 = Concatenate Strings(w3277, w3276, "Fuel Discription :-" ("Substring"), w3287, w3276, w3298, w3276, "Batch Ref Num :-" ("Substring"), w3273, w3276, " Remarks :- " ("Substring"), w3284, w3276, " Date :- " ("Substring"), w3279, w3276, "Tested By :-" ("Substring"), w3281) -> (w3292:string)
                    "REMARKS" <- w3292
                    n2099 = call <vilib>:"Write Characters To File.vi"("append to file? (new file:F)"=FALSE, "character string"=w3294, "file path (dialog if empty)"=w3260) -> ()  [unwired: 2 in, 1 out]
                    n2100 = call <vilib>:"Write Characters To File.vi"("append to file? (new file:F)"=FALSE, "character string"=w3292, "file path (dialog if empty)"=w3259) -> ()  [unwired: 2 in, 1 out]
                  }
                  frame #2 {
                    n2101 = local write "Cycles elapsed"(0 ("Cycles elapsed")) -> ()
                    n2102 = local write "cyclecount"(0 ("cyclecount")) -> ()
                    n2103 = local write "Save & Continue"(FALSE ("OK")) -> ()
                    n2104 = local write "autostrtflg"(TRUE ("autostrtflg")) -> ()
                    n2105 = local write "Save"(FALSE ("Save")) -> ()
                    n2106 = Get Date/Time In Seconds() -> (seconds since 1Jan1904=w3316:timestamp)
                    n2107 = To Double Precision Float(number=w3316) -> (double precision float=w3315:dbl)
                    n2108 = local write "acq timer"(w3315) -> ()
                    n2109 = One Button Dialog(message="Please ensure sample is mounted properly and machine is ready in all aspects for testing !", button name ("OK")="Ok") -> ()  [unwired: 1 out]
                  }
                  frame #3 {
                    n2110 = stacked-sequence {
                      frame #0 {
                        n2111 = local write "Main Dashboard Buttons"(T1."Dashboard" ("Main Dashboard Buttons")) -> ()
                        n2112 = local write "Main Tab"(T2."Acquire" ("Main Tab")) -> ()
                      }
                      frame #1 {
                        n2113 = local write "EVENT LOG"("" ("EVENT LOG")) -> ()
                      }
                      frame #2 {
                        n2114 = Wait (ms)(milliseconds to wait=u32 50) -> ()  [unwired: 1 out]
                      }
                      frame #3 {
                        n2115 = local read "EVENT LOG"() -> (w3327:string)
                        n2116 = call "Event Log.vi"("Content"="Test Details", "EVENT LOG"=w3327) -> ("EVENT LOG"=w3326:string)  [unwired: 8 in, 1 out]
                        n2117 = local write "EVENT LOG"(w3326) -> ()
                      }
                      frame #4 {
                        n2118 = Wait (ms)(milliseconds to wait=u32 50) -> ()  [unwired: 1 out]
                      }
                      frame #5 {
                        n2119 = local read "FILE"() -> (w3329:string)
                        n2120 = Concatenate Strings("File Name :" ("Content"), w3329) -> (w3330:string)
                        n2121 = local read "EVENT LOG"() -> (w3333:string)
                        n2122 = call "Event Log.vi"("Content"=w3330, "EVENT LOG"=w3333) -> ("EVENT LOG"=w3332:string)  [unwired: 8 in, 1 out]
                        n2123 = local write "EVENT LOG"(w3332) -> ()
                      }
                      frame #6 {
                        n2124 = Wait (ms)(milliseconds to wait=u32 50) -> ()  [unwired: 1 out]
                      }
                      frame #7 {
                        n2125 = local read "Batch Ref Num :"() -> (w3335:string)
                        n2126 = Concatenate Strings("Batch Ref No :" ("Content"), w3335) -> (w3336:string)
                        n2127 = local read "EVENT LOG"() -> (w3339:string)
                        n2128 = call "Event Log.vi"("Content"=w3336, "EVENT LOG"=w3339) -> ("EVENT LOG"=w3338:string)  [unwired: 8 in, 1 out]
                        n2129 = local write "EVENT LOG"(w3338) -> ()
                      }
                      frame #8 {
                        n2130 = Wait (ms)(milliseconds to wait=u32 50) -> ()  [unwired: 1 out]
                      }
                      frame #9 {
                        n2131 = local read "tested by"() -> (w3341:string)
                        n2132 = Concatenate Strings("Tested By :" ("Content"), w3341) -> (w3342:string)
                        n2133 = local read "EVENT LOG"() -> (w3345:string)
                        n2134 = call "Event Log.vi"("Content"=w3342, "EVENT LOG"=w3345) -> ("EVENT LOG"=w3344:string)  [unwired: 8 in, 1 out]
                        n2135 = local write "EVENT LOG"(w3344) -> ()
                      }
                      frame #10 {
                        n2136 = Wait (ms)(milliseconds to wait=u32 50) -> ()  [unwired: 1 out]
                      }
                      frame #11 {
                        n2137 = local read "TEST STANDARD"() -> (w3348:T3)
                        n2138 = case shown="\"ASTM D6079\", Default" w3348 {
                          tunnel: ["ASTM D6079" "ISO 12156" "CEC F-096-A-06" "Custom"] -> w3347
                          frame "ASTM D6079", Default {
                          }
                          frame "ISO 12156" {
                          }
                          frame "CEC F-096-A-06" {
                          }
                          frame "Custom" {
                          }
                        }
                        n2139 = Concatenate Strings("Test Standard :" ("Content"), w3347) -> (w3349:string)
                        n2140 = local read "EVENT LOG"() -> (w3352:string)
                        n2141 = call "Event Log.vi"("Content"=w3349, "EVENT LOG"=w3352) -> ("EVENT LOG"=w3351:string)  [unwired: 8 in, 1 out]
                        n2142 = local write "EVENT LOG"(w3351) -> ()
                      }
                      frame #12 {
                        n2143 = Wait (ms)(milliseconds to wait=u32 50) -> ()  [unwired: 1 out]
                      }
                      frame #13 {
                        n2144 = local read "Fuel Discription :"() -> (w3358:string)
                        n2145 = Concatenate Strings("Fuel Description :" ("Content"), w3358) -> (w3359:string)
                        n2146 = local read "EVENT LOG"() -> (w3362:string)
                        n2147 = call "Event Log.vi"("Content"=w3359, "EVENT LOG"=w3362) -> ("EVENT LOG"=w3361:string)  [unwired: 8 in, 1 out]
                        n2148 = local write "EVENT LOG"(w3361) -> ()
                      }
                      frame #14 {
                        n2149 = Wait (ms)(milliseconds to wait=u32 50) -> ()  [unwired: 1 out]
                      }
                      frame #15 {
                        n2150 = local read "Remarks :"() -> (w3364:string)
                        n2151 = Concatenate Strings("Remarks :" ("Content"), w3364) -> (w3365:string)
                        n2152 = local read "EVENT LOG"() -> (w3368:string)
                        n2153 = call "Event Log.vi"("Content"=w3365, "EVENT LOG"=w3368) -> ("EVENT LOG"=w3367:string)  [unwired: 8 in, 1 out]
                        n2154 = local write "EVENT LOG"(w3367) -> ()
                      }
                      frame #16 {
                        n2155 = Wait (ms)(milliseconds to wait=u32 50) -> ()  [unwired: 1 out]
                      }
                      frame #17 {
                        n2156 = local read "Operator ID"() -> (w3370:string)
                        n2157 = Concatenate Strings("Operator ID :" ("Content"), w3370) -> (w3372:string)
                        n2158 = local read "EVENT LOG"() -> (w3374:string)
                        n2159 = call "Event Log.vi"("Content"=w3372, "EVENT LOG"=w3374) -> ("EVENT LOG"=w3373:string)  [unwired: 8 in, 1 out]
                        n2160 = local write "EVENT LOG"(w3373) -> ()
                      }
                      frame #18 {
                        n2161 = Wait (ms)(milliseconds to wait=u32 50) -> ()  [unwired: 1 out]
                      }
                      frame #19 {
                        n2162 = local read "EVENT LOG"() -> (w3378:string)
                        n2163 = call "Event Log.vi"("Content"="Test Parameter", "EVENT LOG"=w3378) -> ("EVENT LOG"=w3377:string)  [unwired: 8 in, 1 out]
                        n2164 = local write "EVENT LOG"(w3377) -> ()
                      }
                      frame #20 {
                        n2165 = Wait (ms)(milliseconds to wait=u32 50) -> ()  [unwired: 1 out]
                      }
                      frame #21 {
                        n2166 = local read "Set Hz"() -> (w3382:dbl)
                        n2167 = Number To Fractional String(number=w3382, precision (6)=i16 2) -> (F-format string=w3381:string)  [unwired: 2 in]
                        n2168 = Concatenate Strings("Set Frequency [Hz] :" ("Content"), w3381) -> (w3384:string)
                        n2169 = local read "EVENT LOG"() -> (w3386:string)
                        n2170 = call "Event Log.vi"("Content"=w3384, "EVENT LOG"=w3386) -> ("EVENT LOG"=w3385:string)  [unwired: 8 in, 1 out]
                        n2171 = local write "EVENT LOG"(w3385) -> ()
                      }
                      frame #22 {
                        n2172 = Wait (ms)(milliseconds to wait=u32 50) -> ()  [unwired: 1 out]
                      }
                      frame #23 {
                        n2173 = local read "NORMAL LOAD"() -> (w3389:dbl)
                        n2174 = Number To Fractional String(number=w3389, precision (6)=i16 2) -> (F-format string=w3390:string)  [unwired: 2 in]
                        n2175 = Concatenate Strings("Set Load [N] :" ("Content"), w3390) -> (w3392:string)
                        n2176 = local read "EVENT LOG"() -> (w3394:string)
                        n2177 = call "Event Log.vi"("Content"=w3392, "EVENT LOG"=w3394) -> ("EVENT LOG"=w3393:string)  [unwired: 8 in, 1 out]
                        n2178 = local write "EVENT LOG"(w3393) -> ()
                      }
                      frame #24 {
                        n2179 = Wait (ms)(milliseconds to wait=u32 50) -> ()  [unwired: 1 out]
                      }
                      frame #25 {
                        n2180 = local read "Set Strk"() -> (w3397:dbl)
                        n2181 = Number To Fractional String(number=w3397, precision (6)=i16 2) -> (F-format string=w3398:string)  [unwired: 2 in]
                        n2182 = Concatenate Strings("Set Stroke [mm] :" ("Content"), w3398) -> (w3400:string)
                        n2183 = local read "EVENT LOG"() -> (w3402:string)
                        n2184 = call "Event Log.vi"("Content"=w3400, "EVENT LOG"=w3402) -> ("EVENT LOG"=w3401:string)  [unwired: 8 in, 1 out]
                        n2185 = local write "EVENT LOG"(w3401) -> ()
                      }
                      frame #26 {
                        n2186 = Wait (ms)(milliseconds to wait=u32 50) -> ()  [unwired: 1 out]
                      }
                      frame #27 {
                        n2187 = local read "Set Temp"() -> (w3405:dbl)
                        n2188 = Number To Fractional String(number=w3405, precision (6)=i16 2) -> (F-format string=w3406:string)  [unwired: 2 in]
                        n2189 = Concatenate Strings("Set Temp [deg C] :" ("Content"), w3406) -> (w3408:string)
                        n2190 = local read "EVENT LOG"() -> (w3410:string)
                        n2191 = call "Event Log.vi"("Content"=w3408, "EVENT LOG"=w3410) -> ("EVENT LOG"=w3409:string)  [unwired: 8 in, 1 out]
                        n2192 = local write "EVENT LOG"(w3409) -> ()
                      }
                      frame #28 {
                        n2193 = Wait (ms)(milliseconds to wait=u32 50) -> ()  [unwired: 1 out]
                      }
                      frame #29 {
                        n2194 = local read "Set Rh"() -> (w3413:dbl)
                        n2195 = Number To Fractional String(number=w3413, precision (6)=i16 2) -> (F-format string=w3414:string)  [unwired: 2 in]
                        n2196 = Concatenate Strings("Set Humidity [%RH] :" ("Content"), w3414) -> (w3416:string)
                        n2197 = local read "EVENT LOG"() -> (w3418:string)
                        n2198 = call "Event Log.vi"("Content"=w3416, "EVENT LOG"=w3418) -> ("EVENT LOG"=w3417:string)  [unwired: 8 in, 1 out]
                        n2199 = local write "EVENT LOG"(w3417) -> ()
                      }
                      frame #30 {
                        n2200 = Wait (ms)(milliseconds to wait=u32 50) -> ()  [unwired: 1 out]
                      }
                      frame #31 {
                        n2201 = local read "test time"() -> (w3421:dbl)
                        n2202 = Number To Fractional String(number=w3421, precision (6)=i16 1) -> (F-format string=w3422:string)  [unwired: 2 in]
                        n2203 = Concatenate Strings("Test Time [mins] :" ("Content"), w3422) -> (w3424:string)
                        n2204 = local read "EVENT LOG"() -> (w3426:string)
                        n2205 = call "Event Log.vi"("Content"=w3424, "EVENT LOG"=w3426) -> ("EVENT LOG"=w3425:string)  [unwired: 8 in, 1 out]
                        n2206 = local write "EVENT LOG"(w3425) -> ()
                      }
                    }
                  }
                }
              }
            }
          }
        }
        n2207 = local read "Set Rh"() -> (w2740:dbl)
        n2208 = Add(x=w2741, y=w2766) -> (x+y=w2767:dbl)
        n2209 = Subtract(x=w2741, y=w2766) -> (x-y=w2768:dbl)
        n2210 = Add(x=w2739, y=w2760) -> (x+y=w2761:dbl)
        n2211 = Subtract(x=w2739, y=w2760) -> (x-y=w2762:dbl)
        n2212 = And(x=w2771, y=w2772) -> (x .and. y?=w2770:bool)
        n2213 = Greater Or Equal?(x=w2734, y=15.0) -> (x >= y?=w2735:bool)
        "powstat" <- w2735
        n2214 = local read "Humidity ( %RH )"() -> (w2737:dbl)
        n2215 = case shown="True" w2770 {
          frame False {
            n2216 = local write "tfalg"(0.0 ("tfalg")) -> ()
          }
          frame True {
            n2217 = local read "tfalg"() -> (w2915:dbl)
            n2218 = Equal?(x=w2915, y=0.0) -> (x = y?=w2916:bool)
            n2219 = case shown="True" w2916 {
              frame False {
              }
              frame True {
                n2220 = local read "Total No. of Tests"() -> (w2919:dbl)
                n2221 = local write "tfalg"(1.0 ("tfalg")) -> ()
                n2222 = local write "acq 2"(FALSE ("acq 2")) -> ()
                n2223 = Wait (ms)(milliseconds to wait=u32 200) -> ()  [unwired: 1 out]
                n2224 = Increment(x=w2919) -> (x+1=w2918:dbl)
                n2225 = local write "Total No. of Tests"(w2918) -> ()
              }
            }
          }
        }
        n2226 = In Range and Coerce(upper limit=w2767, x=w2738, lower limit=w2768) -> (In Range?=w2757:bool)  [unwired: 1 out]
        n2227 = Add(x=w2740, y=w2765) -> (x+y=w2764:dbl)
        n2228 = Subtract(x=w2740, y=w2765) -> (x-y=w2763:dbl)
        n2229 = local read "TEMP"() -> (w2736:dbl)
        n2230 = local write "Test \nStatus"(w2776) -> ()
        n2231 = local write "st enable"(w2776) -> ()
        n2232 = local write "PWR"(w2776) -> ()
        n2233 = local write "Save"(w2776) -> ()
        n2234 = local read "Main Tab"() -> (w2733:T2)
        n2235 = case shown="True" w2757 {
          tunnel: [FALSE ("RUN") TRUE ("RUN")] -> w2756
          tunnel: [_ 1] -> w2749
          frame False {
          }
          frame True {
          }
        }
        n2236 = In Range and Coerce(upper limit=w2764, x=w2737, lower limit=w2763) -> (In Range?=w2755:bool)  [unwired: 1 out]
        n2237 = In Range and Coerce(upper limit=w2761, x=w2736, lower limit=w2762) -> (In Range?=w2753:bool)  [unwired: 1 out]
        n2238 = case shown="True" w2769 {
          frame False {
            n2239 = local read "Rt 3"() -> (w2897:bool)
            n2240 = case shown="True" w2897 {
              frame False {
              }
              frame True {
                n2241 = local write "Rt 3"(FALSE ("Rt 3")) -> ()
                n2242 = local write "Json End Flg"(TRUE ("Upld AR 2")) -> ()
              }
            }
            "Rt" <- TRUE ("Rt")
            "Rt 2" <- FALSE ("Rt")
          }
          frame True {
            n2243 = local read "Rt"() -> (w2904:bool)
            n2244 = local write "Rt 2"(TRUE ("Rt 2")) -> ()
            n2245 = case shown="True" w2904 {
              frame False {
              }
              frame True {
                w2905 = TRUE ("Upld AR 2")
                n2246 = local write "Rt"(FALSE ("Rt")) -> ()
                n2247 = local write "Upld AR"(w2905) -> ()
                n2248 = local write "Json St Flg"(w2905) -> ()
              }
            }
            "Rt 3" <- TRUE ("Rt 3")
          }
        }
        n2249 = case shown="True" w2755 {
          tunnel: [FALSE ("RUN") TRUE ("RUN")] -> w2754
          tunnel: [_ 2] -> w2748
          frame False {
          }
          frame True {
          }
        }
        n2250 = case shown="True" w2753 {
          tunnel: [FALSE ("RUN") TRUE ("RUN")] -> w2752
          tunnel: [_ 3] -> w2747
          frame False {
          }
          frame True {
          }
        }
